vi "InitControl.vi"(8 "Force Manual":bool, 11 "Box":bool[](array[boolean])) -> (1 "Manual":bool)   [LabVIEW 2014]
panel:
  in  "Joystick":bool[](array[boolean])
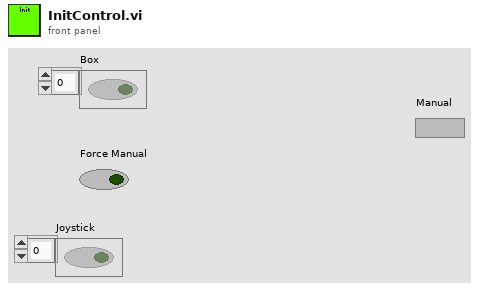
[diagram p1: front panel]
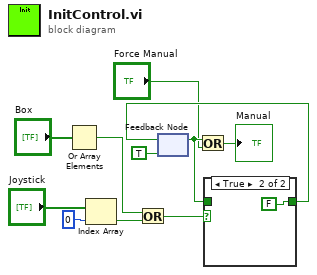
[diagram p0: block diagram]
diagram:
  n1 = Or Array Elements(Boolean array="Box") -> (logical OR=w5:bool)
  n2 = Index Array(array="Joystick", index=0) -> (element=w1:bool)
  n3 = Or(x=w5, y=w1) -> (x .or. y?=w4:bool)
  n4 = feedback #1(TRUE) -> (w9:bool)
  n5 = Or(x=w9, y="Force Manual") -> (x .or. y?=→"Manual":bool)
  n6 = case shown="True" w4 {
    tunnel: w9 -> [w12 _]
    tunnel: [w12 FALSE] -> w10
    frame False {
    }
    frame True {
    }
  }
  n7 = feedback-in #1(w10) -> ()
